vi "Formata_Numeros.vi"(1 "Formato ex-> 7.2":string="7.2", 2 "Valor num":string=" 281.52") -> (0 "resulting string":string)   [LabVIEW 2018]
panel:
  # "7.2"
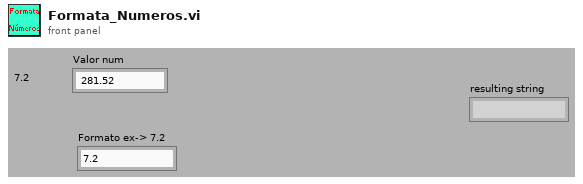
[diagram p1: front panel]
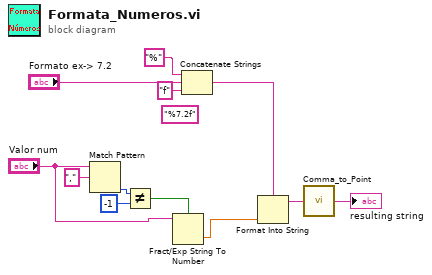
[diagram p0: block diagram]
diagram:
  (unwired) "%7.2f" ("format string")
  n1 = Match Pattern(string="Valor num", regular expression=",") -> (offset past match=w5:i32)  [unwired: 1 in, 3 out]
  n2 = Not Equal?(x=w5, y=-1) -> (x != y?=w3:bool)
  n3 = Fract/Exp String To Number(use system decimal point (T)=w3, string="Valor num") -> (number=w11:dbl)  [unwired: 2 in, 1 out]
  n4 = Concatenate Strings("%", "Formato ex-> 7.2", "f" ("string")) -> (w7:string)
  n5 = Format Into String(format string=w7, w11) -> (resulting string=w12:string)  [unwired: 2 in, 1 out]
  n6 = call "Comma_to_Point.vi"("Lat_A"=w12) -> ("Saída"=→"resulting string":string)
